vi "make_arbitrary_stimulus.vi"(4 "Trace controls":T2[](array[typedef])=[{"+ stim"=FALSE, "Relative"=FALSE, "Scale"=enum."1X", "Probe point"=enum."Position (tip)", "XYZ selector"={"Boolean"=FALSE, "Boolean 2"=FALSE, "Boolean 3"=FALSE}, "To tip"=FALSE}, {"+ stim"=FALSE, "Relative"=FALSE, "Scale"=enum."1X", "Probe point"=enum."Position (tip)", "XYZ selector"={"Boolean"=FALSE, "Boolean 2"=FALSE, "Boolean 3"=FALSE}, "To tip"=FALSE}, {"+ stim"=FALSE, "Relative"=FALSE, "Scale"=enum."1X", "Probe point"=enum."Position (tip)", "XYZ selector"={"Boolean"=FALSE, "Boolean 2"=FALSE, "Boolean 3"=FALSE}, "To tip"=FALSE}, {"+ stim"=FALSE, "Relative"=FALSE, "Scale"=enum."1X", "Probe point"=enum."Position (tip)", "XYZ selector"={"Boolean"=FALSE, "Boolean 2"=FALSE, "Boolean 3"=FALSE}, "To tip"=FALSE}], 6 "Signal file path":path, 10 "Parameters":sgl[](array[numeric]) format="%#_4p", 11 "Kind":T1) -> (3 "Stimulus":sgl[][](array[numeric]))   [LabVIEW 2012]
uses:
  arb_stimulus_kind.ctl
  Trace controls.ctl
  probe_point.ctl
  <vilib>/Analysis/3filter.llb/Chebyshev Filter (DBL).vi
  <vilib>/Utility/file.llb/Read From Spreadsheet File (DBL).vi
  <vilib>/Analysis/NI_AALBase.lvlib
panel:
  # "Alternative step function with zero DC offset that starts and ends at zero.  May be more suitable to spectral analyis."
  # "Length (sec)"
  # "Stimulus is read from a file (on the real-time target.)  Each line in the file is a single stimulus sample, with up to six floating point numbers (space delimited.)"
  # "Swept-sine signal (chirp) where frequency is an exponential function of time"
  # "Length (sec)"
  # "Low corner (Hz)"
  # "High corner (Hz)"
  # "Band-limited Gaussian noise."
  # "Length (sec)"
  # "Low corner (Hz)"
  # "High corner (Hz)"
  # "Spiral with linear spacing (Archimedes) and constant linear velocity."
  # "Radius (mm)"
  # "Spacing (mm)"
  # "Linear vel (mm/sec)"
  # "Store trace data into stimulus.  Handle KF state may be replayed as \"Total pose\" stimulus."
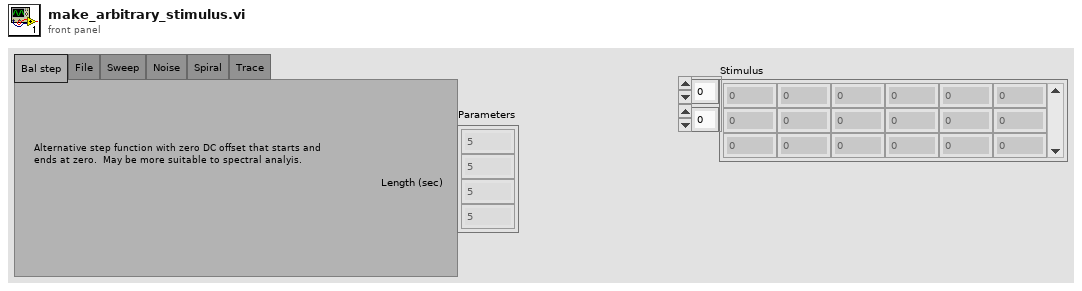
[diagram p1: front panel]
types:
  T1 = typedef "arb_stimulus_kind.ctl" = enum32{"Bal step", "File", "Sweep", "Noise", "Spiral", "Trace"}
  T2 = typedef "Trace controls.ctl" = cluster{"+ stim":bool, "Relative":bool, "Scale":enum16{"1X", "10X", "100X", "1KX", "10KX"}, "Probe point":T3, "XYZ selector":cluster{"Boolean":bool, "Boolean 2":bool, "Boolean 3":bool}, "To tip":bool}
  T3 = typedef "probe_point.ctl" = enum16{"Position (tip)", "Position (RCM)", "Null pos (tip)", "Null pos (RCM)", "V limiter (tip)", "V Limiter (RCM)", "Goal (tip)", "Goal (RCM)", "Link pos 0", "Link pos 1", "KF link pos 0", "KF link pos 1", "Link rate 0", "Link rate 1", "Link residue 0", "Link residue 1", "Link goal 0", "Link goal 1", "Rate limit 0", "Rate limit 1", "Link error 0", "Link error 1", "Controller 0", "Controller 1", "Output 0", "Output 1", "Drive 0", "Drive 1", "Stimulus 0", "Stimulus 1", "Trace data 0", "Trace data 1", "Analog data 0", "Analog data 1", "Status flags", "Light 0", "Light 1", "Light 2", "Light 3", "Light 4", "Light 5", "Goal origin", "Goal rotation 0", "Goal rotation 1", "Goal rotation 2", "Output origin", "Output rotation 0", "Output rotation 1", "Output rotation 2", "Handle origin", "Handle rotation 0", "Handle rotation 1", "Handle rotation 2", "Handle position", "Handle velocity", "Handle acceleration", "Handle angles", "Handle angle rates", "Handle pos residue", "Handle angle residue", "Trace length"}
  T4 = enum32{"Lowpass", "Highpass", "Bandpass", "Bandstop"}
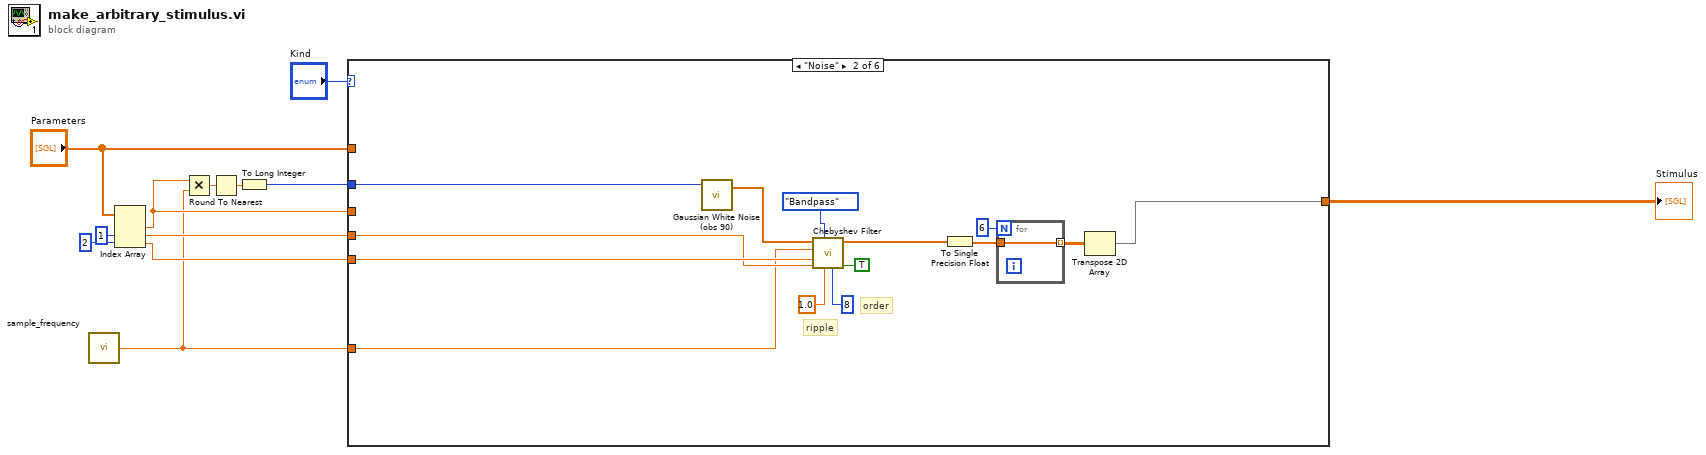
[diagram p0: block diagram]
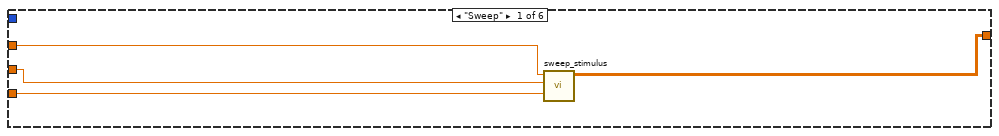
[diagram p2: hidden frame]
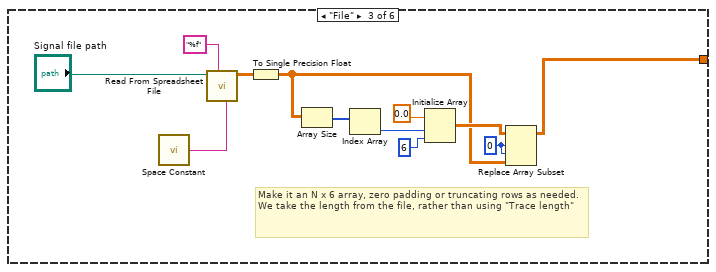
[diagram p3: hidden frame]
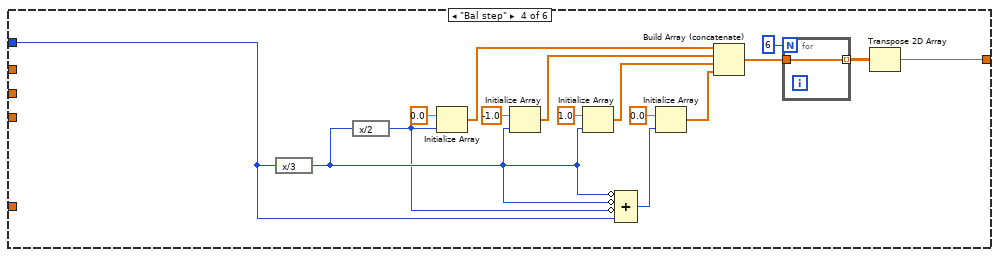
[diagram p4: hidden frame]
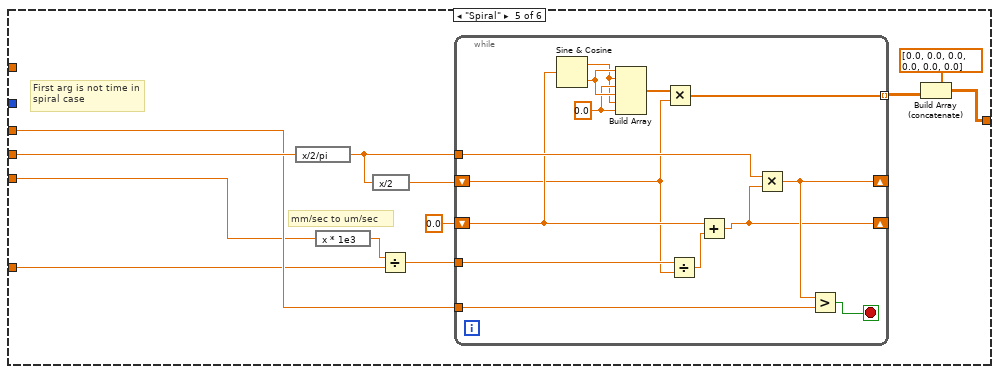
[diagram p5: hidden frame]
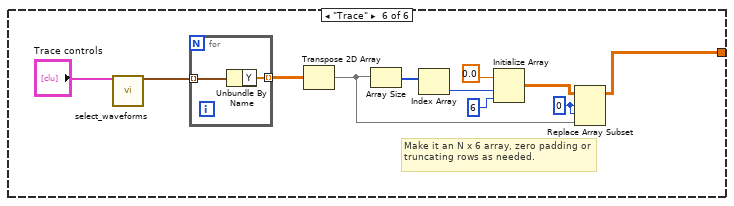
[diagram p6: hidden frame]
diagram:
  n1 = call "sample_frequency.vi"() -> ("Sample frequency"=w1:dbl)
  n2 = Index Array(array="Parameters", index #2=1 ("index"), index #3=2 ("index")) -> (element #1=w3:sgl, element #2=w6:sgl, element #3=w5:sgl)  [unwired: 1 in]
  n3 = Multiply(x=w3, y=w1) -> (x*y=w10:dbl)
  n4 = Round To Nearest(number=w10) -> (nearest integer value=w11:dbl)
  n5 = To Long Integer(number=w11) -> (32bit integer=w12:i32)
  n6 = case shown="\"Noise\"" "Kind" {
    tunnel: w12 -> [_ w30 _ w49 _ _]
    tunnel: w6 -> [w14 w26 _ _ w71 _]
    tunnel: w5 -> [w13 w27 _ _ w63 _]
    tunnel: [w16 w21 w33 w50 w64 w87] -> w2
    tunnel: "Parameters" -> [_ _ _ _ _ _]
    tunnel: w3 -> [w15 _ _ _ w69 _]
    tunnel: w1 -> [_ w17 _ _ w61 _]
    frame "Sweep" {
      n7 = call "sweep_stimulus.vi"("High corner (Hz)"=w13, "Low corner (Hz)"=w14, "Length (sec)"=w15) -> ("Result"=w16:sgl[][])  [unwired: 8 in]
    }
    frame "Noise" {
      # "order"
      # "ripple"
      n8 = call <vilib>:"Gaussian White Noise (obs 90).vi"("samples"=w30) -> ("Gaussian noise pattern"=w28:dbl[])  [unwired: 2 in, 1 out]
      n9 = call-poly <vilib>:"Chebyshev Filter.vi"("init/cont (init:F)"=TRUE, "order"=8, "ripple(dB)"=1.0, "filter type"=T4."Bandpass", "low cutoff freq: fl"=w26, "high cutoff freq: fh"=w27, "sampling freq: fs"=w17, "X"=w28) -> ("Filtered X"=w22:dbl[])  [unwired: 3 out]
      n10 = To Single Precision Float(number=w22) -> (single precision float=w19:sgl[])
      n11 = for {
        N: 6 -> [_]
        tunnel: w19 -> [w31]
        tunnel: [w31] -> w18 mode=indexing
      }
      n12 = Transpose 2D Array(2D array=w18) -> (transposed array=w21:sgl[][])
    }
    frame "File" {
      w35 = 0 ("index (row)")
      # "Make it an N x 6 array, zero padding or truncating rows as needed.  We take the length from the file, rather than using \"Trace length\""
      n13 = call <vilib>:"Space Constant.vi"() -> ("String"=w42:string)
      n14 = call-poly <vilib>:"Read From Spreadsheet File.vi"("delimiter (\\t)"=w42, "format (%.3f)"="%f", "file path (dialog if empty)"="Signal file path") -> ("all rows"=w43:dbl[][])  [unwired: 2 in, 6 out]
      n15 = To Single Precision Float(number=w43) -> (single precision float=w34:sgl[][])
      n16 = Array Size(array=w34) -> (size(s)=w39:i32[])
      n17 = Index Array(array=w39) -> (element=w37:i32)  [unwired: 1 in]
      n18 = Initialize Array(sgl 0.0, w37, 6 ("dimension size")) -> (w36:sgl[][])
      n19 = Replace Array Subset(array=w36, new element=w34, index (row)=w35, index (col)=w35) -> (w33:sgl[][])
    }
    frame "Bal step" {
      n20 = expression code="x/3"(w49) -> (w48:i32)
      n21 = expression code="x/2"(w48) -> (w47:i32)
      n22 = Initialize Array(sgl 0.0 ("element"), w47) -> (w54:sgl[])
      n23 = Initialize Array(sgl -1.0 ("element"), w48) -> (w53:sgl[])
      n24 = Initialize Array(sgl 1.0 ("element"), w48) -> (w52:sgl[])
      n25 = Compound Arithmetic op=ADD(invert w48, invert w48, invert w47, w49) -> (w55:i32)
      n26 = Initialize Array(sgl 0.0 ("element"), w55) -> (w51:sgl[])
      n27 = Build Array (concatenate)(w54, w53, w52, w51) -> (w45:sgl[])
      n28 = for {
        N: 6 -> [_]
        tunnel: w45 -> [w60]
        tunnel: [w60] -> w44 mode=indexing
      }
      n29 = Transpose 2D Array(2D array=w44) -> (transposed array=w50:sgl[][])
    }
    frame "Spiral" {
      # "First arg is not time in spiral case"
      # "mm/sec to um/sec"
      n30 = expression code="x/2/pi"(w71) -> (w67:sgl)
      n31 = expression code="x * 1e3"(w63) -> (w62:sgl)
      n32 = expression code="x/2"(w67) -> (w68:sgl)
      n33 = Divide(x=w62, y=w61) -> (x/y=w70:dbl)
      n34 = while {
        tunnel: w67 -> [w86]
        shift-right: [w73] -> _
        shift-left: sgl 0.0 ("element") -> [w82]
        tunnel: w70 -> [w80]
        tunnel: w69 -> [w84]
        shift-right: [w83] -> _
        shift-left: w68 -> [w79]
        tunnel: [w78] -> w65 mode=indexing
        stop <- w85 stop-if-true
        w75 = sgl 0.0 ("cos(x)")
        n35 = Sine & Cosine(0:w82) -> (1:w74:dbl, 2:w76:dbl)
        n36 = Build Array(w76, w74, w75, w76, w74, w75) -> (w77:dbl[])
        n37 = Multiply(x=w77, y=w79) -> (x*y=w78:dbl[])
        n38 = Divide(x=w80, y=w79) -> (x/y=w81:dbl)
        n39 = Add(x=w82, y=w81) -> (x+y=w73:dbl)
        n40 = Multiply(x=w86, y=w73) -> (x*y=w83:dbl)
        n41 = Greater?(x=w83, y=w84) -> (0:w85:bool)
      }
      n42 = Build Array (concatenate)(sgl[] [0.0, 0.0, 0.0, 0.0, 0.0, 0.0] ("Parameters"), w65) -> (w64:dbl[][])
    }
    frame "Trace" {
      w89 = 0 ("index (row)")
      # "Make it an N x 6 array, zero padding or truncating rows as needed."
      n43 = call "select_waveforms.vi"("Trace controls"="Trace controls") -> ("Waveforms out"=w96:waveform(sgl)[])  [unwired: 11 in, 3 out]
      n44 = for {
        tunnel: w96 -> [w99] mode=indexing
        tunnel: [w98] -> w95 mode=indexing
        n45 = Unbundle By Name(w99) -> ("Y"=w98:sgl[])
      }
      n46 = Transpose 2D Array(2D array=w95) -> (transposed array=w88:sgl[][])
      n47 = Array Size(array=w88) -> (size(s)=w93:i32[])
      n48 = Index Array(array=w93) -> (element=w91:i32)  [unwired: 1 in]
      n49 = Initialize Array(sgl 0.0, w91, 6 ("dimension size")) -> (w90:sgl[][])
      n50 = Replace Array Subset(array=w90, new element=w88, index (row)=w89, index (col)=w89) -> (w87:sgl[][])
    }
  }
  "Stimulus" <- w2
